vi "求导.vi"() -> ()   [LabVIEW 2018]
uses:
  <vilib>/Analysis/NI_AALPro.lvlib
panel:
  in  "停止":bool
  out "结果":dbl[](array[numeric])
  in  "X":dbl[](array[numeric])
  in  "method":u16(ring) caption="方法" items=["二阶中心", "四阶中心", "前向", "后向"]
  in  "dt":dbl=1.0 format="%0.2f"
  in  "Final Condition":dbl[](array[numeric])=[0.0] caption="最终条件" format="%#_6f"
  in  "Initial Condition":dbl[](array[numeric])=[0.0] caption="初始条件" format="%#_6f"
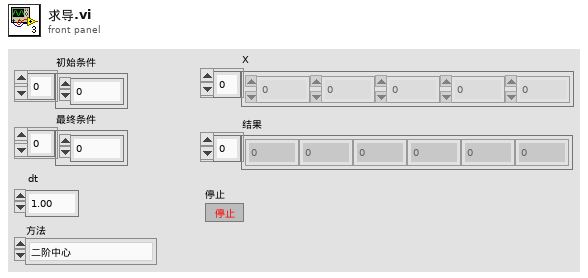
[diagram p1: front panel]
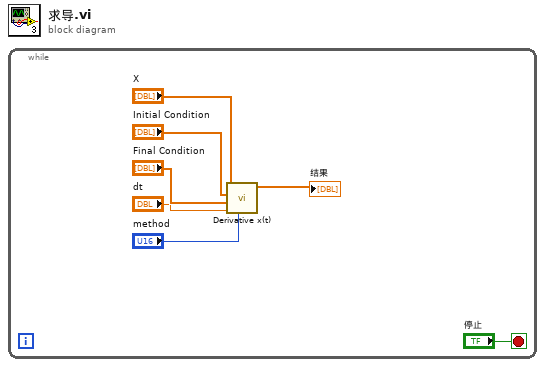
[diagram p0: block diagram]
diagram:
  n1 = while {
    stop <- "停止" stop-if-true
    n2 = call <vilib>:"Derivative x(t).vi"("method"="method", "dt"="dt", "Final Condition"="Final Condition", "Initial Condition"="Initial Condition", "X"="X") -> ("dX/dt"=→"结果":dbl[])  [unwired: 5 in, 1 out]
  }
